vi "圆整到2的N次方(Boolean).vi"(1 "Integer":i32) -> (0 "Power of 2 Integer":i32)   [LabVIEW 2012]
doc: "Round up to a power of two.\n\nAuthored by David A Moore\nsupport@mooregoodideas.com\nwww.mooregoodideas.com\n\nCopyright (c) 2010, Moore Good Ideas, Inc.\n\nAll rights reserved.\n\nRedistribution and use in source and binary forms, with or without modification, are permitted provided that the following conditions are met:\n\n * Redistributions of source code must retain the above copyright notice, this list of conditions and the following disclaimer.\n * Redistributions in binary form must reproduce the above copyright notice, this list of conditions and the following disclaimer in the documentation and/or other materials provided with the distribution.\n * Neither the name of Moore Good Ideas, Inc. nor the names of its contributors may be used to endorse or promote products derived from this software without specific prior written permission.\n\nTHIS SOFTWARE IS PROVIDED BY THE COPYRIGHT HOLDERS AND CONTRIBUTORS \"AS IS\" AND ANY EXPRESS OR IMPLIED WARRANTIES, INCLUDING, BUT NOT LIMITED TO, THE IMPLIED WARRANTIES OF MERCHANTABILITY AND FITNESS FOR A PARTICULAR PURPOSE ARE DISCLAIMED. IN NO EVENT SHALL THE COPYRIGHT OWNER OR CONTRIBUTORS BE LIABLE FOR ANY DIRECT, INDIRECT, INCIDENTAL, SPECIAL, EXEMPLARY, OR CONSEQUENTIAL DAMAGES (INCLUDING, BUT NOT LIMITED TO, PROCUREMENT OF SUBSTITUTE GOODS OR SERVICES; LOSS OF USE, DATA, OR PROFITS; OR BUSINESS INTERRUPTION) HOWEVER CAUSED AND ON ANY THEORY OF LIABILITY, WHETHER IN CONTRACT, STRICT LIABILITY, OR TORT (INCLUDING NEGLIGENCE OR OTHERWISE) ARISING IN ANY WAY OUT OF THE USE OF THIS SOFTWARE, EVEN IF ADVISED OF THE POSSIBILITY OF SUCH DAMAGE."
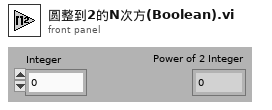
[diagram p1: front panel]
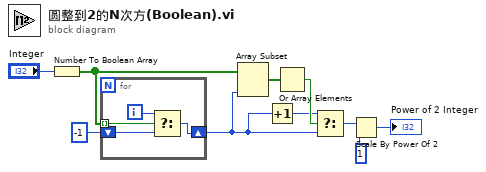
[diagram p0: block diagram]
diagram:
  n1 = Number To Boolean Array(number="Integer") -> (Boolean array=w9:bool[])
  n2 = for {
    tunnel: w9 -> [w14] mode=indexing
    shift-right: [w11] -> w7
    shift-left: -1 -> [w12]
    i -> [w13]
    n3 = Select(t=w13, s=w14, f=w12) -> (s? t:f=w11:i32)
  }
  n4 = Array Subset(array=w9, length=w7) -> (w5:bool[])  [unwired: 1 in]
  n5 = Increment(x=w7) -> (x+1=w2:i32)
  n6 = Or Array Elements(Boolean array=w5) -> (logical OR=w3:bool)
  n7 = Select(t=w2, s=w3, f=w7) -> (s? t:f=w1:i32)
  n8 = Scale By Power Of 2(n=w1, x=1 ("Power of 2 Integer")) -> (x*2^n=→"Power of 2 Integer":i32)
